vi "DashboardGetProgramState.vi"(8 "Dashboard":refnum<k24>, 11 "error in":errorcluster) -> (0 "Response":cluster{"Message":string, "Succeed":bool}, 1 "State":i32(ring) items=["Stopped", "Playing", "Paused"], 2 "Name":string, 3 "error out":errorcluster)   [LabVIEW 2022 SP3, in "UnderAutomation.UniversalRobots.lvlib"]
uses:
  UnderAutomation.UniversalRobots.lvlib
  C:/Users/fg/Documents/UniversalRobots.vi/LabVIEW_2023/UnderAutomation.UniversalRobots/lib/UnderAutomation.UniversalRobots.dll
  LabVIEW_2023/UnderAutomation.UniversalRobots/lib/UnderAutomation.UniversalRobots.dll
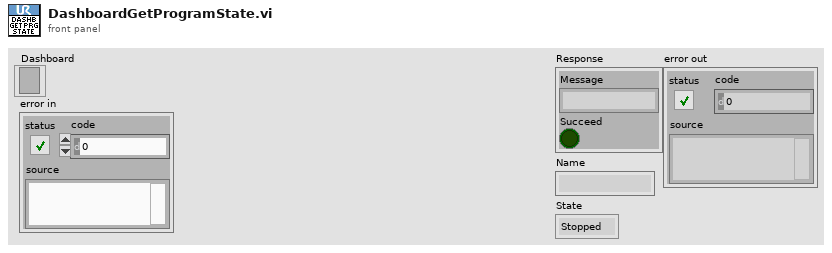
[diagram p1: front panel]
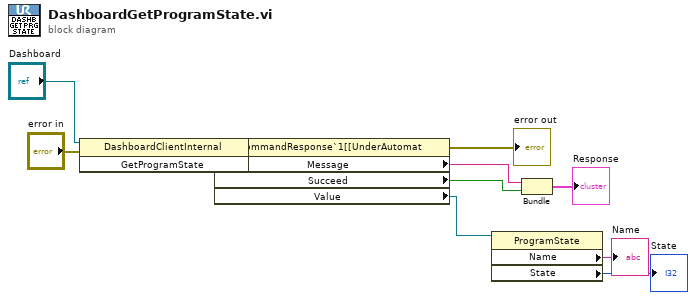
[diagram p0: block diagram]
diagram:
  n1 = invoke class="DashboardClientInternal" method="GetProgramState"(reference="Dashboard", error in="error in") -> (error out=w5:errorcluster, "GetProgramState"=w10:refnum<k24>)  [unwired: 1 in, 1 out]
  n2 = property class="CommandResponse`1[[UnderAutomat"(reference=w10, error in=w5) -> (error out=→"error out":errorcluster, "Message"=w9:string, "Succeed"=w8:bool, "Value"=w3:refnum<k24>)  [unwired: 1 out]
  n3 = property class="ProgramState"(reference=w3) -> ("Name"=→"Name":string, "State"=→"State":i32)  [unwired: 1 in, 2 out]
  n4 = Bundle("Message"=w9, "Succeed"=w8) -> (→"Response":cluster{"Message":string, "Succeed":bool})  [unwired: 1 in]
